vi "OPC UA Client-Read.vi"() -> ()   [LabVIEW 2017]
uses:
  <vilib>/OPCUA/client/internal/Read Double.vi
  <vilib>/OPCUA/NI OPC UA Client.lvlib
panel:
  in  "Item Path":string="Process Data.Temperature"
  in  "Stop Button":bool
  out "Temperature Value":dbl
  in  "Server Endpoint URL":string="opc.tcp://XPS15HPH:49580"
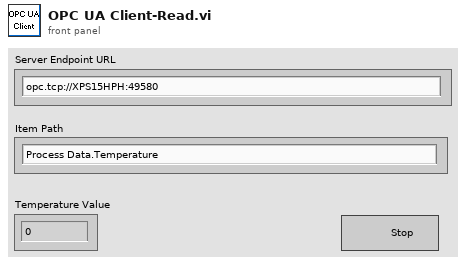
[diagram p1: front panel]
types:
  T1 = cluster{"message mode":enum16{"None", "Sign", "Sign and Encrypt"}, "security":enum16{"Basic256", "Basic128Rsa15"}}
  T2 = typedef "OPC UA Client Refnum.ctl" = refnum<k21>
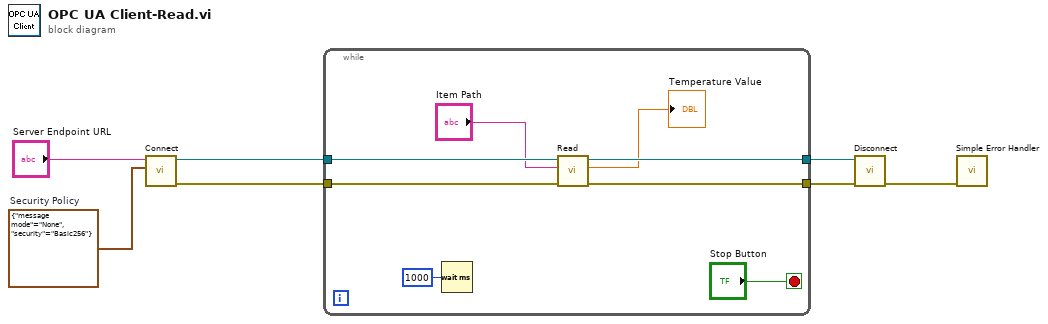
[diagram p0: block diagram]
diagram:
  w1 = T1 {"message mode"=enum."None", "security"=enum."Basic256"}  # Security Policy
  n1 = call <vilib>:"Connect.vi"("security policy"=w1, "server endpoint URL"="Server Endpoint URL") -> ("error out"=w6:errorcluster, "OPC UA client refnum out"=w7:T2)  [unwired: 7 in, 1 out]
  n2 = while {
    tunnel: w7 -> [w13]
    tunnel: w6 -> [w12]
    tunnel: [w11] -> w5
    tunnel: [w10] -> w3
    stop <- "Stop Button" stop-if-true
    n3 = Wait (ms)(milliseconds to wait=u32 1000) -> ()  [unwired: 1 out]
    n4 = call-poly <vilib>:"Read.vi"("error in (no error)"=w12, "node ID"="Item Path", "OPC UA client refnum in"=w13) -> ("error out"=w10:errorcluster, "value"=→"Temperature Value":dbl, "OPC UA client refnum out"=w11:T2)  [unwired: 4 in, 2 out]
  }
  n5 = call <vilib>:"Disconnect.vi"("error in (no error)"=w3, "OPC UA client refnum in"=w5) -> ("error out"=w4:errorcluster)  [unwired: 9 in]
  n6 = call <vilib>:"Simple Error Handler.vi"("error in (no error)"=w4) -> ()  [unwired: 4 in, 5 out]
